vi "CropImageARGB.vi"(7 "Origin (Default: 0,0)":T1, 8 "error in (no error)":errorcluster, 9 "Cropped Size":T2, 10 "ARGB Image Destination":refnum<data-value>, 11 "ARGB Image Source":refnum<data-value>) -> (0 "error out":errorcluster, 3 "ARGB Image Destination (duplicate)":refnum<data-value>)   [LabVIEW 2020, in "g_ar_toolkit.image.lvlib"]
uses:
  g_ar_toolkit.image.lvlib
  g_ar_toolkit.common/Image Size (Integer).ctl
  g_ar_toolkit.common/Image Point (Integer).ctl
  <vilib>/Utility/error.llb/Error Cluster From Error Code.vi
  2dc01dea-48f6-4df4-8727-934e95e7e307.vi
  g_ar_toolkit.common/g_ar_toolkit_common.lvlib
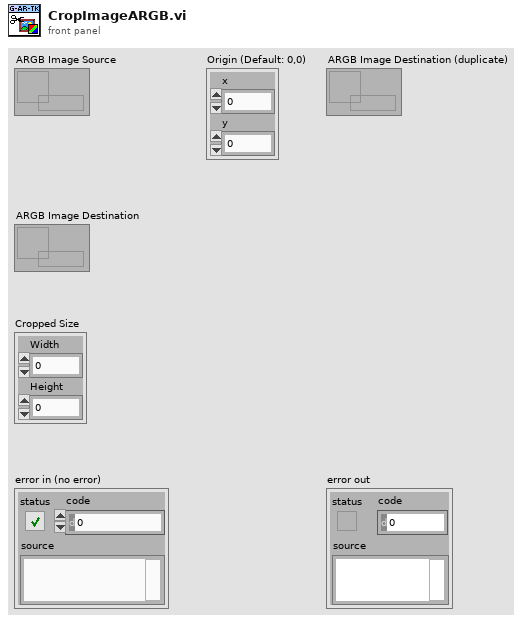
[diagram p1: front panel]
types:
  T1 = typedef "g_ar_toolkit_common.lvlib/Image Point (Integer).ctl" = cluster{"x":i32, "y":i32}
  T2 = typedef "g_ar_toolkit_common.lvlib/Image Size (Integer).ctl" = cluster{"Width":u16, "Height":u16}
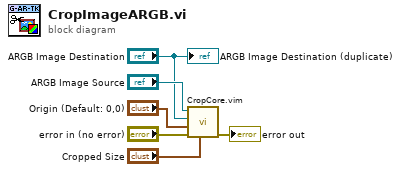
[diagram p0: block diagram]
diagram:
  n1 = call "CropCore.vim"("Size"="Cropped Size", "error in (no error)"="error in (no error)", "Origin"="Origin (Default: 0,0)", "Dst"="ARGB Image Destination", "Src"="ARGB Image Source") -> ("error out"=→"error out":errorcluster)  [unwired: 6 in]
  "ARGB Image Destination (duplicate)" <- "ARGB Image Destination"
